vi "4_mation_lab_view.vi"() -> ()   [LabVIEW 2021]
panel:
  in  "VISA resource name":refnum<visa-resource-name>
  out "Temp Chart":dbl(graph)
  in  "Table Control":string[][](table)
  out "Temparature":dbl(slide) scale=0.0..100.0
  out "Temp":bool
  out "Intruder":bool
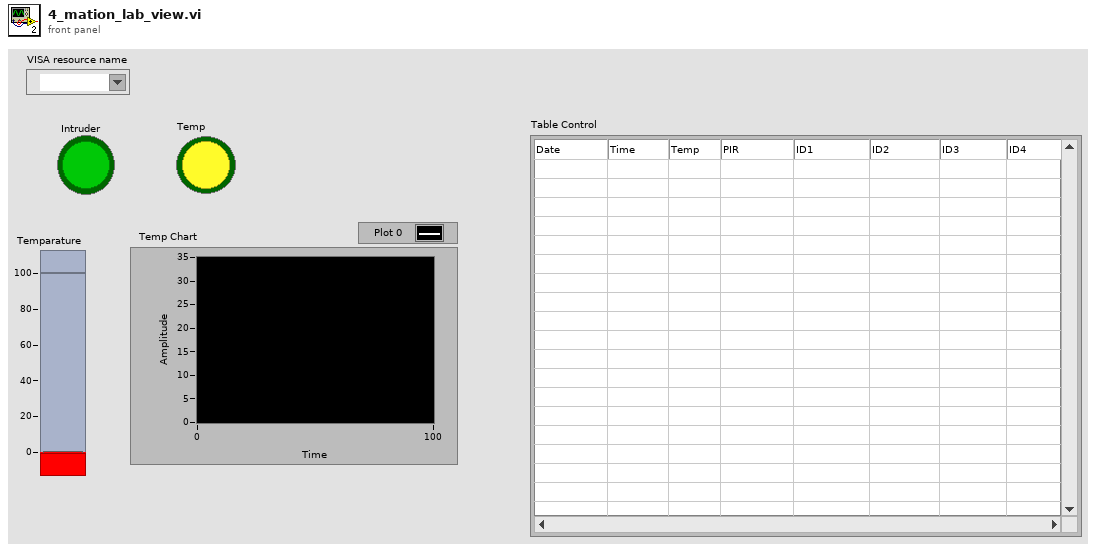
[diagram p1: front panel]
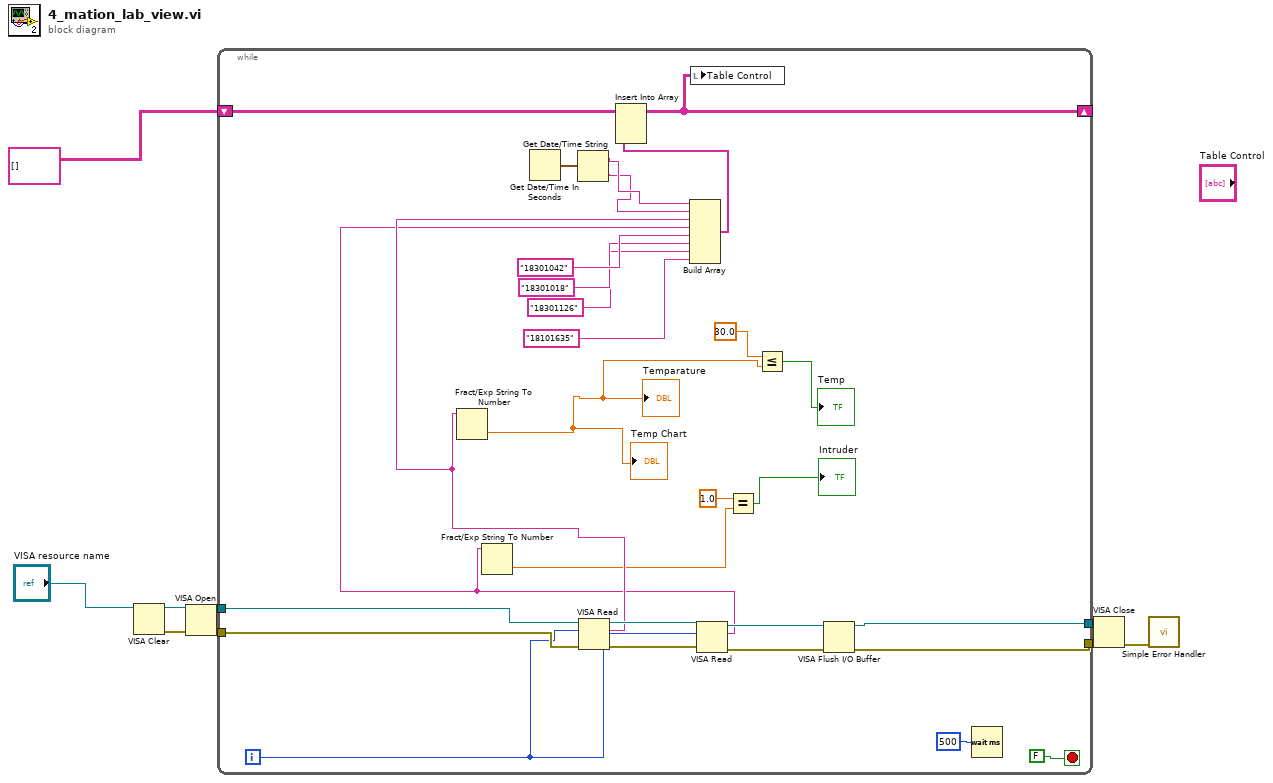
[diagram p0: block diagram]
diagram:
  n1 = VISA Clear(VISA resource name="VISA resource name") -> (VISA resource name out=w8:refnum<visa-resource-name>, error out=w9:errorcluster)  [unwired: 1 in]
  n2 = VISA Open(error in (no error)=w9, VISA resource name=w8) -> (VISA resource name=w6:refnum<visa-resource-name>, error out=w5:errorcluster)  [unwired: 3 in]
  n3 = while {
    tunnel: w6 -> [w38]
    tunnel: w5 -> [w37]
    tunnel: [w34] -> w3
    tunnel: [w31] -> w4
    shift-right: [w16] -> _
    shift-left: string[][] [] -> [w28]
    i -> [w30]
    stop <- FALSE stop-if-true
    n4 = Get Date/Time In Seconds() -> (seconds since 1Jan1904=w27:timestamp)
    n5 = Get Date/Time String(seconds (now)=w27) -> (date string=w26:string, time string=w25:string)  [unwired: 2 in]
    n6 = VISA Read(VISA resource name=w38, byte count=w30, error in (no error)=w37) -> (VISA resource name out=w36:refnum<visa-resource-name>, read buffer=w24:string, error out=w33:errorcluster)  [unwired: 1 out]
    n7 = Fract/Exp String To Number(string=w24) -> (number=w11:dbl)  [unwired: 3 in, 1 out]
    "Temparature" <- w11
    "Temp Chart" <- w11
    n8 = VISA Read(VISA resource name=w36, byte count=w30, error in (no error)=w33) -> (VISA resource name out=w35:refnum<visa-resource-name>, read buffer=w23:string, error out=w32:errorcluster)  [unwired: 1 out]
    n9 = Fract/Exp String To Number(string=w23) -> (number=w14:dbl)  [unwired: 3 in, 1 out]
    n10 = Build Array(w26, w25, w24, w23, "18301042" ("element"), "18301018" ("element"), "18301126" ("element"), "18101635" ("element")) -> (w18:string[])
    n11 = Insert Into Array(array=w28, new element=w18) -> (w16:string[][])  [unwired: 2 in]
    n12 = local write "Table Control"(w16) -> ()
    n13 = Equal?(x=1.0, y=w14) -> (x = y?=→"Intruder":bool)
    n14 = Less Or Equal?(x=30.0, y=w11) -> (x <= y?=→"Temp":bool)
    n15 = VISA Flush I/O Buffer(VISA resource name=w35, error in (no error)=w32) -> (VISA resource name out=w34:refnum<visa-resource-name>, error out=w31:errorcluster)  [unwired: 1 in]
    n16 = Wait (ms)(milliseconds to wait=u32 500) -> ()  [unwired: 1 out]
  }
  n17 = VISA Close(VISA resource name=w3, error in (no error)=w4) -> (error out=w7:errorcluster)
  n18 = call <vilib>:"Simple Error Handler.vi"("error in (no error)"=w7) -> ()  [unwired: 4 in, 5 out]
